vi "Old WT500 Read Power.vi"(0 "VISA resource name":refnum<visa-resource-name>="WT500", 1 "WT500 CMDS":T1, 5 "V Range (8: 1000V)":u16(ring)=6 items=["AUTO", "15", "30", "60", "100", "150", "300", "600", "1000", "7.5", "15", "30", "50", "75", "150", "300", "500"], 7 "I Range (7: 40A)":u16(ring)=7 items=["AUTO", "500 mA", "1 A", "2 A", "5 A", "10 A", "20 A", "40 A", "S-AUTO", "50 mV", "100 mV", "200 mV", "500 mV", "1 V", "2 V", "5 V", "10 V", "250 mA", "500 mA", "1 A", "2.5 A", "5 A", "10 A", "20 A", "25 mV", "50 mV", "100 mV", "250 mV", "500 mV", "1 V", "2.5 V", "5 V"], 11 "error in (no error)":errorcluster) -> (4 "VISA resource name out":refnum<visa-resource-name>="WT500", 6 "PowerData":T2={"Current L1"=236.2, "Current L2"=17.749, "Power"=4192.0, "WattHours"=0.0}, 10 "Measurement Values":dbl[](array[numeric]) format="%.4p", 14 "Label":string[](array[string])=["Urms:Element 1", "Urms:Element 2", "Irms:Element 1", "Irms:Element 2", "P:Sigma", "Wp:Sigma", "I +peak:Element 1", "I +peak:Element 2"], 15 "error out":errorcluster)   [LabVIEW 2016]
uses:
  Type Definitions/WT500 Dryer Power Data.ctl
  Type Definitions/WT500 Sequences.ctl
  LLBs/ykwt500.llb/YKWT500 Configure Numeric Item (Set).vi
panel:
  out "(Max Current)":dbl
  in  "Pole":u16(ring)=1 items=["NONE", "Element 1", "Element 2", "Element 3", "Sigma"]
  in  "Measurement":u16(ring)=1 items=["None", "Urms", "Umn", "Udc", "Urmn", "Uac", "Irms", "Imn", "Idc", "Irmn", "Iac", "P", "S", "Q", "Lambda", "Phi", "Freq U", "Freq I", "U +peak", "U -peak", "I +peak", "I -peak", "Cf U", "Cf I", "Time", "Wp", "Wp+", "Wp-", "q", "q+", "q-", "WS", "WQ", "Eta 1", "Eta 2", "F1", "F2", "F3", "F4", "F5", "F6", "F7", "F8", "U(k)", "I(k)", "P(k)", "S(k)", "Q(k)", "Lambda(k)", "Phi(k)", "Phi U(k)", "Phi I(k)", "Uhdf(k)", "Ihdf(k)", "Phdf(k)", "Uthd", "Ithd", "Pthd", "Phi Ui-Uj", "Phi Ui-Uk", "Phi Ui-Ii", "Phi Ui-Ij", "Phi Ui-Ik", "Delta 1", "Delta 2", "Delta 3", "Delta 4"]
  out "Data Length":i32
  out "Read Data":string
  in  "Write Data":string
  out "Scan Error":bool
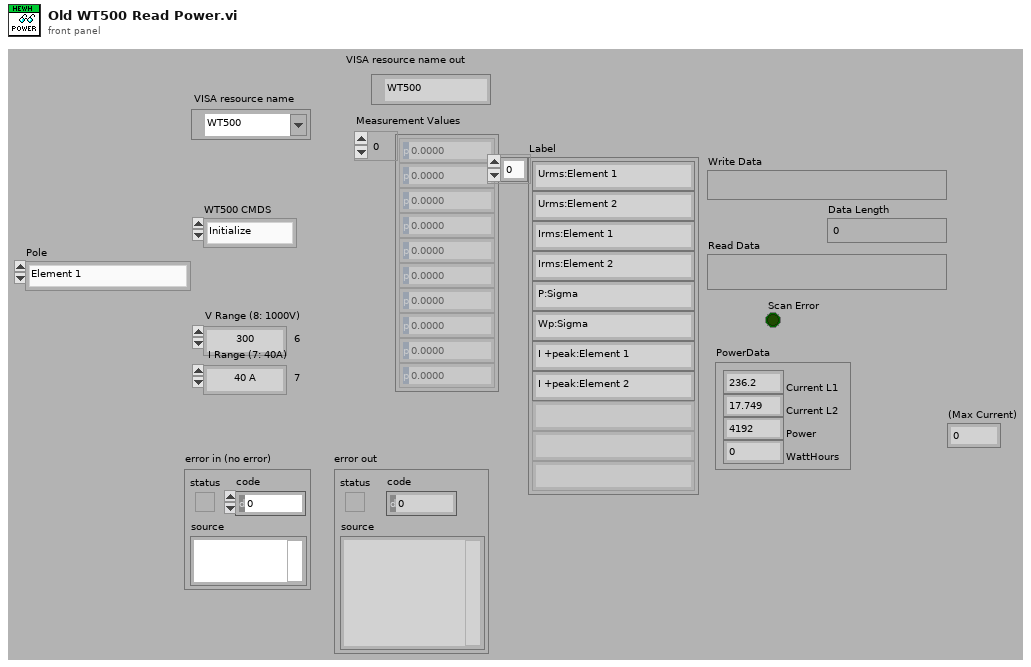
[diagram p1: front panel]
types:
  T1 = typedef "WT500 Sequences.ctl" = enum16{"Initialize", "GetReadings", "GetErrors", "Close", "NoOp", "MiscCmd"}
  T2 = typedef "WT500 Dryer Power Data.ctl" = cluster{"Current L1":dbl, "Current L2":dbl, "Power":dbl, "WattHours":dbl}
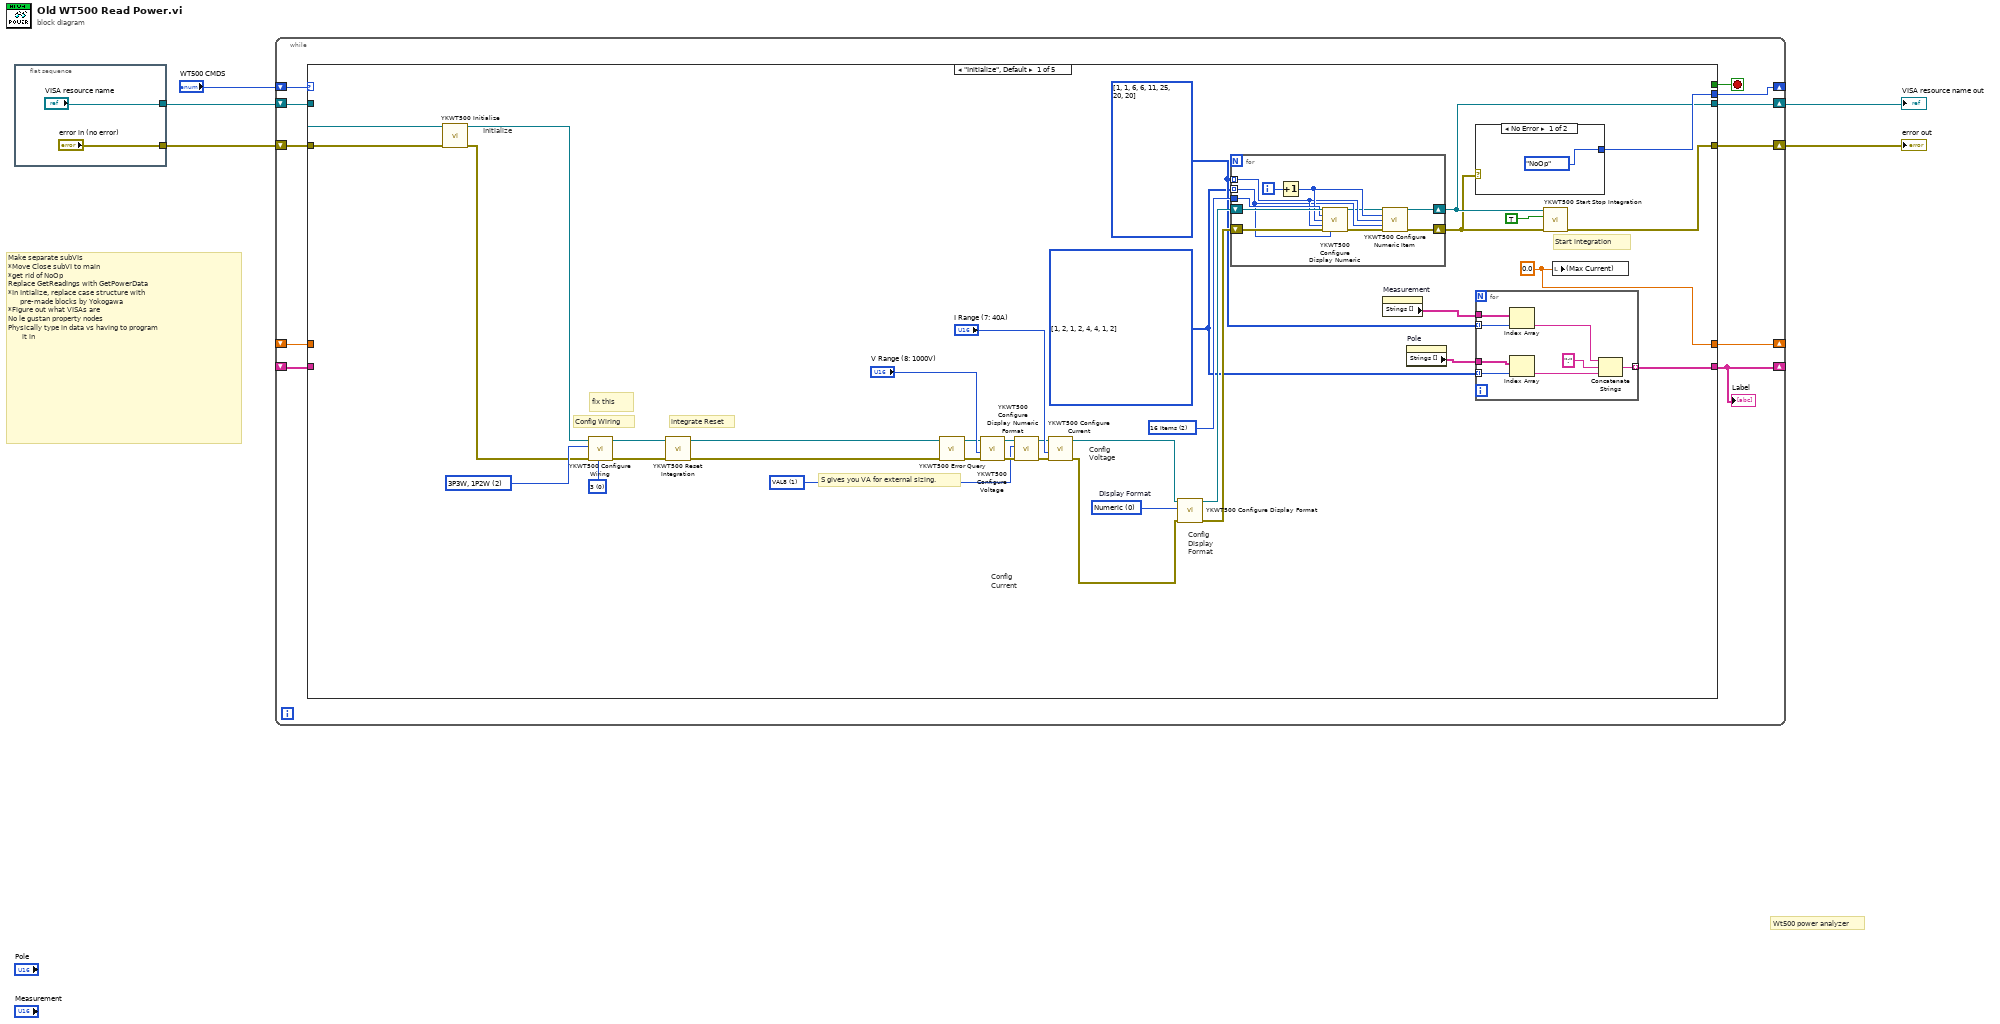
[diagram p0: block diagram]
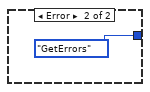
[diagram p2: hidden frame]
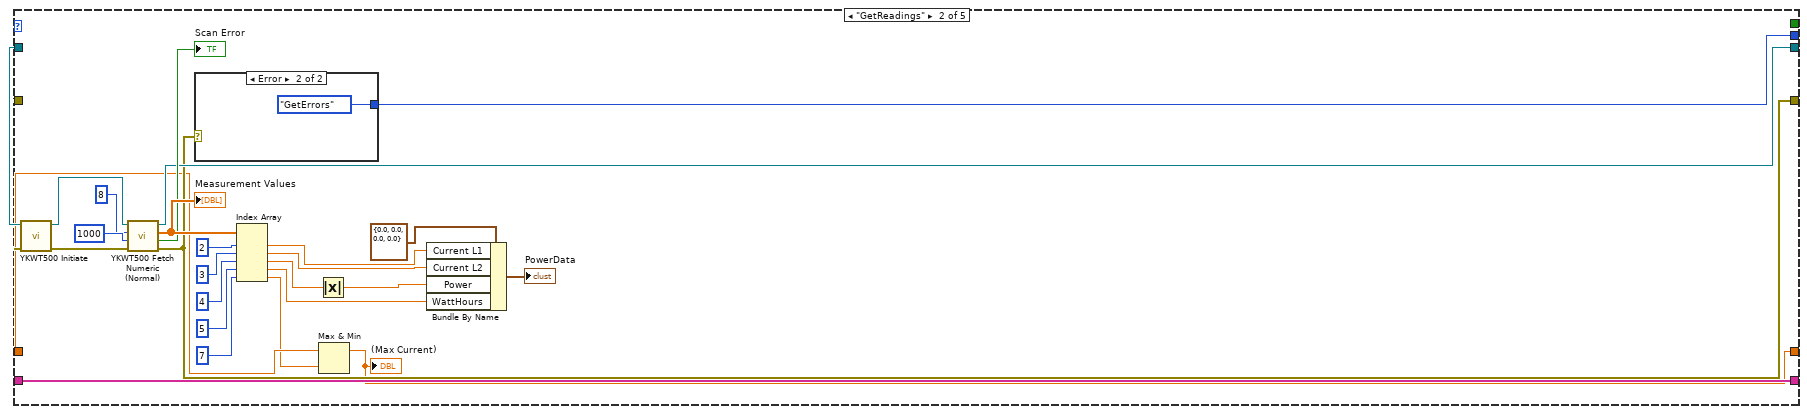
[diagram p3: hidden frame]
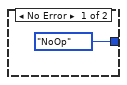
[diagram p4: hidden frame]
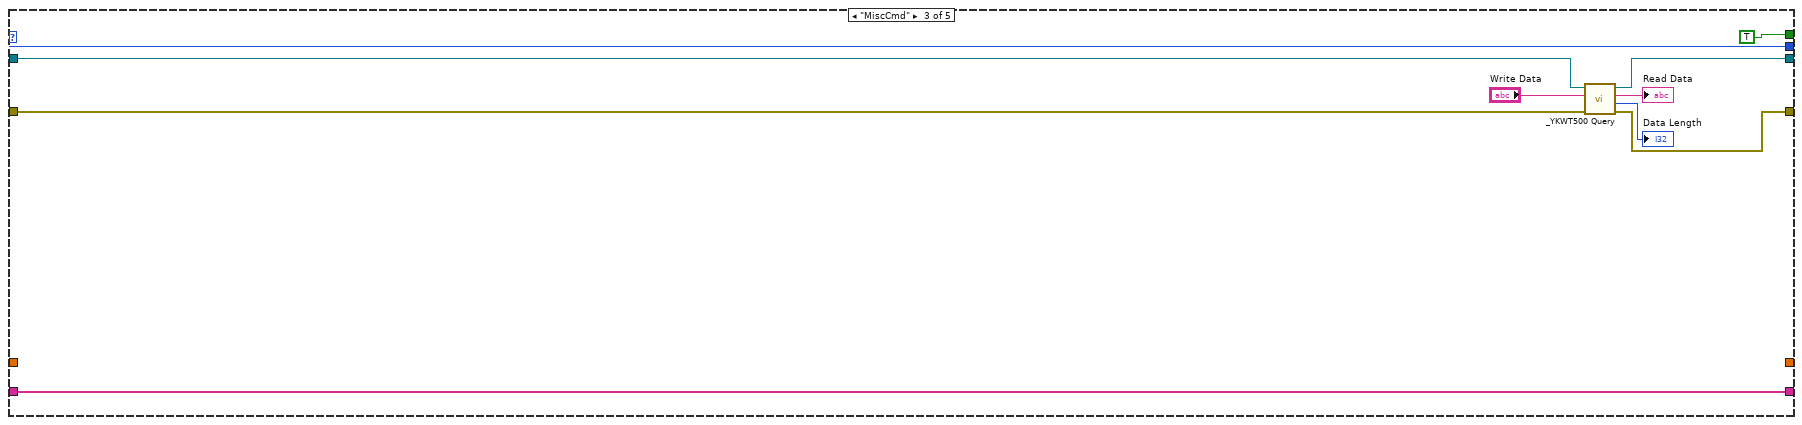
[diagram p5: hidden frame]
diagram:
  # "Make separate subVIs \n*Move Close subVI to main\n*get rid of NoOp\nReplace GetReadings with GetPowerData\n*In Intialize, replace case structure with\n      pre-made blocks by Yokogawa\n*Figure out what VISAs are\nNo le gustan property nodes\nPhysically type in data vs having to program\n       it in"
  # "Wt500 power analyzer"
  n1 = flat-sequence {
    tunnel: ["error in (no error)"] -> w2
    tunnel: ["VISA resource name"] -> w1
    frame #0 {
    }
  }
  n2 = while {
    shift-right: [w16] -> w4
    shift-left: w2 -> [w17]
    shift-right: [w14] -> _
    shift-left: "WT500 CMDS" -> [w18]
    shift-right: [w12] -> w3
    shift-left: w1 -> [w13]
    shift-right: [w10] -> _
    shift-left: _ -> [w11]
    shift-right: [w9] -> _
    shift-left: _ -> [w8]
    stop <- w15 stop-if-true
    n3 = case shown="\"Initialize\", Default" w18 {
      selector: w18 -> [_ _ w113 w115 w124]
      tunnel: w17 -> [w49 w83 w110 w118 w122]
      tunnel: [w22 w86 w109 w118 w122] -> w16
      tunnel: [_ _ TRUE _ _] -> w15
      tunnel: [w48 w85 w113 w115 w124] -> w14
      tunnel: w13 -> [w47 w84 w112 w119 w123]
      tunnel: [w21 w87 w111 w119 w123] -> w12
      tunnel: [w36 w80 w105 w116 w120] -> w10
      tunnel: w11 -> [_ w80 w105 w116 w120]
      tunnel: [w35 w76 _ w117 w121] -> w9
      tunnel: w8 -> [_ w78 _ w117 w121]
      frame "Initialize", Default {
        w29 = u16 0 items=["3", "6"] ("Crest Factor (0: 3)")
        w30 = u16 2 items=["1P2W, 1P2W, 1P2W", "1P3W, 1P2W", "3P3W, 1P2W", "1P2W, 1P3W", "1P2W, 3P3W", "3P4W", "3V3A"] ("Wiring (0: 1P2W, 1P2W, 1P2W)")
        w31 = u16[] [1, 2, 1, 2, 4, 4, 1, 2] items=["NONE", "Element 1", "Element 2", "Element 3", "Sigma"]
        w32 = u16[] [1, 1, 6, 6, 11, 25, 20, 20] items=["None", "Urms", "Umn", "Udc", "Urmn", "Uac", "Irms", "Imn", "Idc", "Irmn", "Iac", "P", "S", "Q", "Lambda", "Phi", "Freq U", "Freq I", "U +peak", "U -peak", "I +peak", "I -peak", "Cf U", "Cf I", "Time", "Wp", "Wp+", "Wp-", "q", "q+", "q-", "WS", "WQ", "Eta 1", "Eta 2", "F1", "F2", "F3", "F4", "F5", "F6", "F7", "F8", "U(k)", "I(k)", "P(k)", "S(k)", "Q(k)", "Lambda(k)", "Phi(k)", "Phi U(k)", "Phi I(k)", "Uhdf(k)", "Ihdf(k)", "Phdf(k)", "Uthd", "Ithd", "Pthd", "Phi Ui-Uj", "Phi Ui-Uk", "Phi Ui-Ii", "Phi Ui-Ij", "Phi Ui-Ik", "Delta 1", "Delta 2", "Delta 3", "Delta 4"] ("Array of Measurements")
        w35 = 0.0
        w39 = u16 1 items=["VAL4", "VAL8", "VAL16", "MATRIX", "ALL"] ("Display Format (0: Numeric)")
        w44 = u16 2 items=["4 Items", "8 Items", "16 Items", "Matrix"] ("Numeric Format (0: 4 Items)")
        w54 = u16 0 items=["Numeric", "Wave", "Bar", "Vector", "Trend"]  # Display Format
        # "fix this"
        # "Start integration"
        # "integrate Reset"
        # "Config Wiring"
        # "S gives you VA for external sizing."
        # "Config\nDisplay\nFormat"
        # "Config\nCurrent"
        # "Config\nVoltage"
        # "Initialize"
        n4 = call "YKWT500 Initialize.vi"("error in (no error)"=w49, "VISA resource name"=w47) -> ("error out"=w28:errorcluster, "VISA resource name out"=w19:refnum<visa-resource-name>)  [unwired: 7 in, 1 out]
        n5 = call "YKWT500 Configure Wiring.vi"("Crest Factor (0: 3)"=w29, "error in (no error)"=w28, "Wiring (0: 1P2W, 1P2W, 1P2W)"=w30, "VISA resource name"=w19) -> ("error out"=w27:errorcluster, "VISA resource name out"=w26:refnum<visa-resource-name>)  [unwired: 6 in]
        n6 = call "YKWT500 Reset Integration.vi"("error in (no error)"=w27, "VISA resource name"=w26) -> ("error out"=w24:errorcluster, "VISA resource name out"=w25:refnum<visa-resource-name>)  [unwired: 8 in]
        n7 = call "YKWT500 Error Query.vi"("error in (no error)"=w24, "VISA resource name"=w25) -> ("error out"=w33:errorcluster, "VISA resource name out"=w34:refnum<visa-resource-name>)  [unwired: 6 in, 2 out]
        n8 = call "YKWT500 Configure Voltage.vi"("error in (no error)"=w33, "Voltage Range (8: 1000V)"="V Range (8: 1000V)", "VISA resource name"=w34) -> ("error out"=w43:errorcluster, "VISA resource name out"=w40:refnum<visa-resource-name>)  [unwired: 7 in]
        n9 = call "YKWT500 Configure Display Numeric Format.vi"("error in (no error)"=w43, "Numeric Format (0: 4 Items)"=w39, "VISA resource name"=w40) -> ("error out"=w42:errorcluster, "VISA resource name out"=w41:refnum<visa-resource-name>)  [unwired: 7 in]
        n10 = call "YKWT500 Configure Current.vi"("error in (no error)"=w42, "Current Range (7: 40A)"="I Range (7: 40A)", "VISA resource name"=w41) -> ("error out"=w53:errorcluster, "VISA resource name out"=w52:refnum<visa-resource-name>)  [unwired: 7 in]
        n11 = call "YKWT500 Configure Display Format.vi"("error in (no error)"=w53, "Display Format (0: Numeric)"=w54, "VISA resource name"=w52) -> ("error out"=w45:errorcluster, "VISA resource name out"=w46:refnum<visa-resource-name>)  [unwired: 7 in]
        n12 = for {
          shift-right: [w65] -> w21
          shift-left: w46 -> [w73]
          shift-right: [w63] -> w20
          shift-left: w45 -> [w72]
          tunnel: w44 -> [w70]
          tunnel: w31 -> [w67] mode=indexing
          tunnel: w32 -> [w68] mode=indexing
          i -> [w71]
          n13 = Increment(x=w71) -> (x+1=w69:i32)
          n14 = call "YKWT500 Configure Display Numeric.vi"("VISA resource name"=w73, "Numeric Format (0: 4 Items)"=w70, "Numeric Item Number (1)"=w69, "Numeric Function (0: None)"=w68, "error in (no error)"=w72, "Element (1: Element 1)"=w67) -> ("VISA resource name out"=w66:refnum<visa-resource-name>, "error out"=w64:errorcluster)  [unwired: 8 in]
          n15 = call-poly "YKWT500 Configure Numeric Item.vi"("VISA resource name"=w66, "Numeric Item Number (1)"=w69, "Numeric Function (0: None)"=w68, "Element (1: Element 1)"=w67, "error in (no error)"=w64) -> ("VISA resource name out"=w65:refnum<visa-resource-name>, "error out"=w63:errorcluster)  [unwired: 9 in]
        }
        n16 = property on="Measurement" class="Ring (strict)"() -> ("Strings []"=w38:string[])  [unwired: 2 in, 2 out]
        n17 = property on="Pole" class="Ring (strict)"() -> ("Strings []"=w37:string[])  [unwired: 2 in, 2 out]
        n18 = case shown="No Error" w20 {
          tunnel: [WT500_Sequences."NoOp" ("WT500 CMDS") WT500_Sequences."GetErrors" ("WT500 CMDS")] -> w48
          frame No Error {
          }
          frame Error {
          }
        }
        n19 = for {
          tunnel: w32 -> [w62] mode=indexing
          tunnel: w38 -> [w61]
          tunnel: w31 -> [w60] mode=indexing
          tunnel: w37 -> [w59]
          tunnel: [w55] -> w36 mode=indexing
          n20 = Index Array(array=w61, index=w62) -> (element=w58:string)
          n21 = Index Array(array=w59, index=w60) -> (element=w56:string)
          n22 = Concatenate Strings(w58, ":" ("string"), w56) -> (w55:string)
        }
        n23 = call "YKWT500 Start Stop Integration.vi"("error in (no error)"=w20, "Start/Stop (False: Stop)"=TRUE, "VISA resource name"=w21) -> ("error out"=w22:errorcluster)  [unwired: 7 in, 1 out]
        n24 = local write "(Max Current)"(w35) -> ()
      }
      frame "GetReadings" {
        n25 = call "YKWT500 Initiate.vi"("error in (no error)"=w83, "VISA resource name"=w84) -> ("error out"=w81:errorcluster, "VISA resource name out"=w82:refnum<visa-resource-name>)  [unwired: 8 in]
        n26 = call "YKWT500 Fetch Numeric (Normal).vi"("error in (no error)"=w81, "Timeout (10000 ms)"=u32 1000, "Number of Item (255)"=8, "VISA resource name"=w82) -> ("error out"=w86:errorcluster, "Scan Error"=→"Scan Error":bool, "Measurement Value"=w91:dbl[], "VISA resource name out"=w87:refnum<visa-resource-name>)  [unwired: 4 in]
        "Measurement Values" <- w91
        n27 = case shown="Error" w86 {
          tunnel: [WT500_Sequences."NoOp" ("WT500 CMDS") WT500_Sequences."GetErrors" ("WT500 CMDS")] -> w85
          frame No Error {
          }
          frame Error {
          }
        }
        n28 = Index Array(array=w91, index #1=2 ("index"), index #2=3 ("index"), index #3=4 ("index"), index #4=5 ("index"), index #5=7 ("index")) -> (element #1=w101:dbl, element #2=w100:dbl, element #3=w95:dbl, element #4=w98:dbl, element #5=w77:dbl)
        n29 = Absolute Value(x=w95) -> (abs(x)=w99:dbl)
        n30 = Max & Min(x=w78, y=w77) -> (max(x,y)=w76:dbl)  [unwired: 1 out]
        "(Max Current)" <- w76
        n31 = Bundle By Name(cluster=T2 {"Current L1"=0.0, "Current L2"=0.0, "Power"=0.0, "WattHours"=0.0} ("PowerData"), "Current L1"=w101, "Current L2"=w100, "Power"=w99, "WattHours"=w98) -> (→"PowerData":T2)
      }
      frame "MiscCmd" {
        n32 = call "_YKWT500 Query.vi"("error in (no error)"=w110, "Write Data"="Write Data", "VISA resource name"=w112) -> ("error out"=w109:errorcluster, "Data Length"=→"Data Length":i32, "Read Data"=→"Read Data":string, "VISA resource name out"=w111:refnum<visa-resource-name>)  [unwired: 5 in]
      }
      frame "NoOp" {
      }
      frame "Close" {
      }
    }
    "Label" <- w10
  }
  "error out" <- w4
  "VISA resource name out" <- w3
